vi "Page_Source_Top_Supports_Multiple_Items.vi"(8 "error in (no error)":errorcluster, 11 "AB_PackedLibrary in":refnum<class "AB_PackedLibrary.lvclass">) -> (0 "error out":errorcluster, 2 "multiple items":bool, 3 "AB_PackedLibrary out":refnum<class "AB_PackedLibrary.lvclass">)   [LabVIEW 2020, in "AB_PackedLibrary.lvclass"]
uses:
  <vilib>/AppBuilder/AB_Classes/PackedLib/AB_PackedLibrary.lvclass
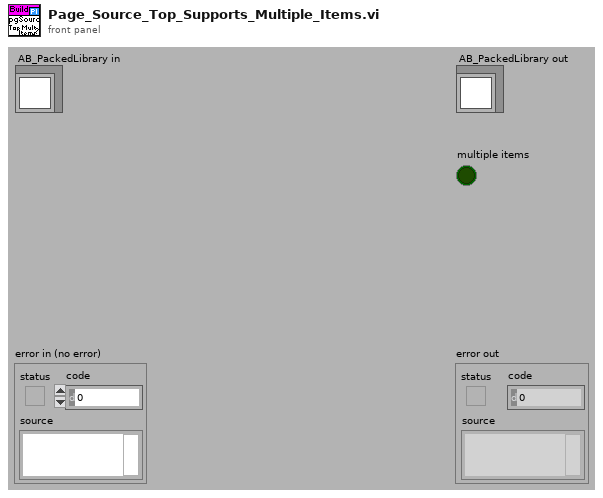
[diagram p1: front panel]
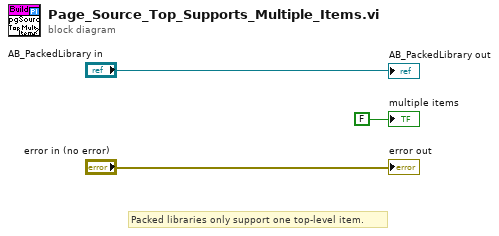
[diagram p0: block diagram]
diagram:
  # "Packed libraries only support one top-level item."
  "error out" <- "error in (no error)"
  "AB_PackedLibrary out" <- "AB_PackedLibrary in"
  "multiple items" <- FALSE ("multiple items")
